vi "Save_Raw_data.vi"(4 "Add to Block Header":string, 7 "append to file? (new file:F)":bool, 8 "Block Timings":T1) -> (2 "Block Header":string)   [LabVIEW 2021]
uses:
  Controls/Block_start_and_end.ctl
  Acquisition/PWA/PWAtasksGLOBAL.vi
  Globals/Meas_global.vi
  Globals/Constants_global.vi
  Globals/LDA_global.vi
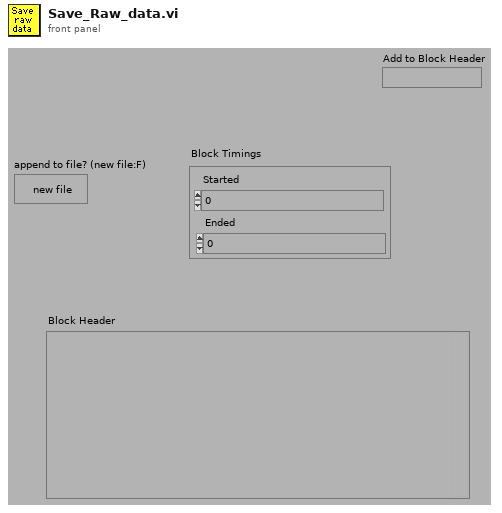
[diagram p1: front panel]
types:
  T1 = typedef "Block_start_and_end.ctl" = cluster{"Started":dbl, "Ended":dbl}
  T2 = cluster{"scale multiplier":dbl, "scale offset":dbl, "Length":i32, "I16 data":i16[], "Sampling rate (Hz)":dbl}
  T3 = typedef "Analysis_info_cluster.ctl" = cluster{"Colour":u32, "Inst type":T4, "Inst name":string, "Symbol":string, "Code name":string, "Extra Info":string, "Inst Array":T5, "Extra Titles":string[], "Extra Values":string[], "U":dbl, "u^2":dbl, "u^3":dbl, "u^4":dbl, "Skew_u":dbl, "Kurt_u":dbl, "Sd Error in Mean":dbl, "% u'/U":dbl, "X":dbl, "Y":dbl, "Z":dbl, "Timescale integral Estimate":dbl, "Sd Error in Variance":dbl, "Calib File":path, "Calib Constants":dbl[], "Output Position":bool, "Stats":enum16{"None", "Basic", "Full"}, "Av Sampling Rate":dbl, "Av No of Samples":dbl, "Total Meas Time (s)":dbl, "ADAM Ch Name":string, "Max value":dbl, "Min value":dbl, "Req Sample Rate Hz":dbl, "Sync Delay Time (s)":dbl, "Ch No":i16, "Device":string, "Use Latest Calib":bool, "Port":string, "Metadata Ch Names":string[], "Metadata Ch Values":string[], "Label":string}
  T4 = typedef "Inst_type.ctl" = enum16{"Raw voltage", "Raw with zero offsetting", "Propeller anemometer", "Pressure Transducer", "Pitot-static tube", "Hot wire", "Cross wire 1", "Cross wire 2", "Generic Linear", "Generic Polynomial", "Generic BackPoly", "Fast FID", "Thermocouple", "Cold wire", "Pulsed Wire", "LDA Vel", "LDA Tran time", "LDA Arr time", "Microphone"}
  T5 = typedef "Instrument_Array.ctl" = enum16{"PWA", "LDA", "Analogue"}
  T6 = typedef "Time_Trace_Cluster.ctl" = cluster{"Weighting":dbl[], "Time (s)":dbl[], "Voltage":dbl[], "Eng Values":dbl[]}
  T7 = cluster{"scale multiplier":dbl, "scale offset":dbl}[]
  T8 = typedef "PWA_Data.ctl" = enum16{"No PWA Data", "One Ch PWA"}
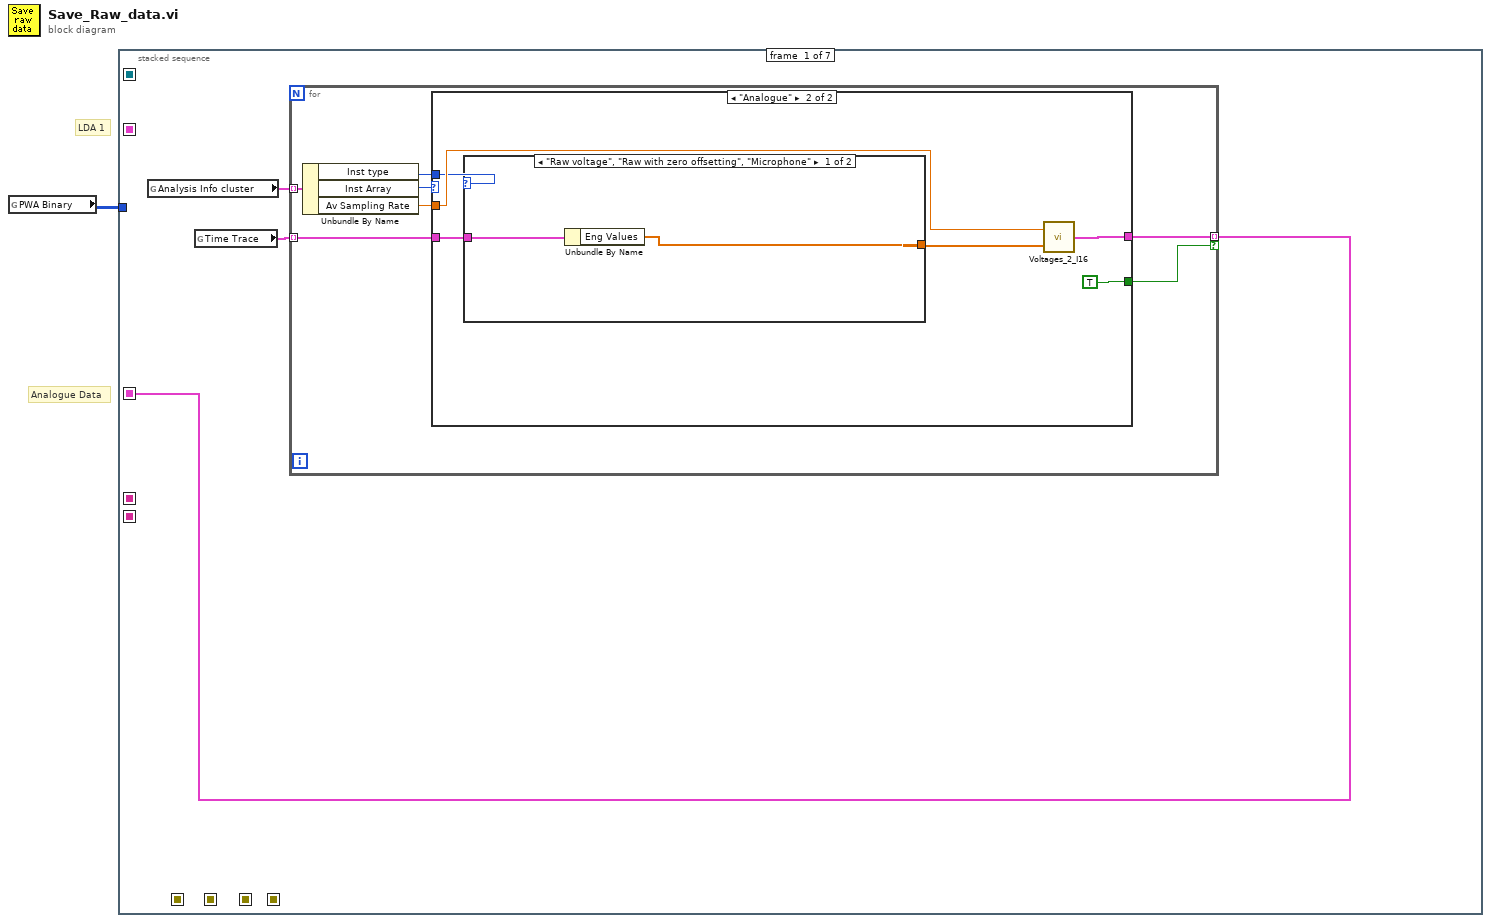
[diagram p0: block diagram]
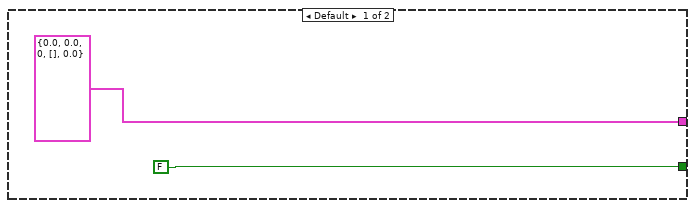
[diagram p2: hidden frame]
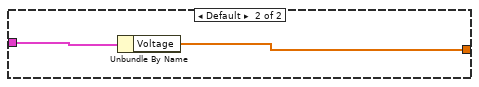
[diagram p3: hidden frame]
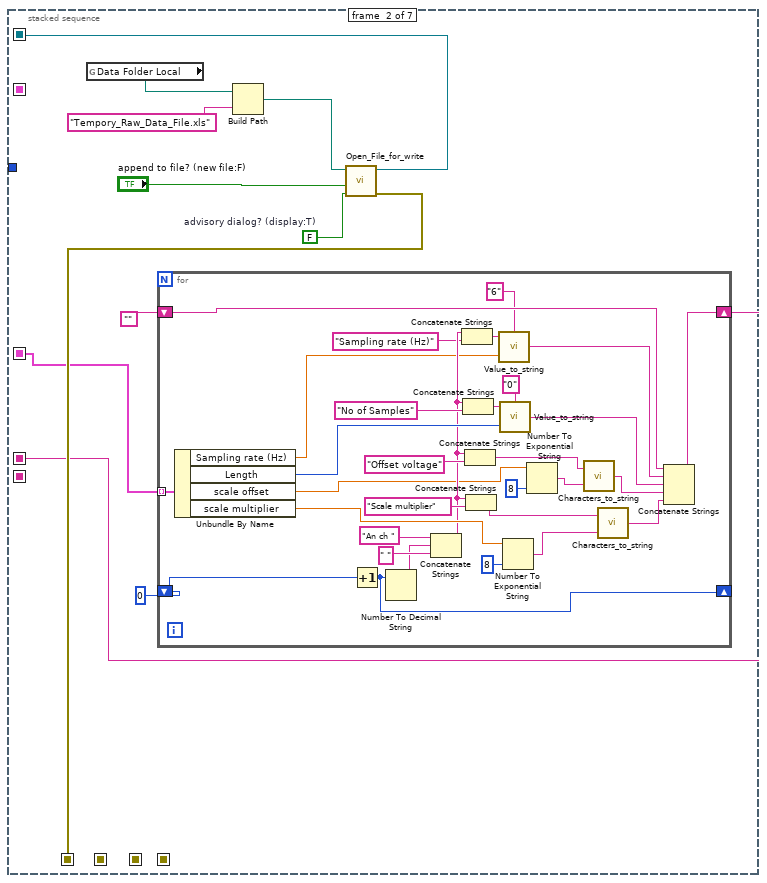
[diagram p4: hidden frame]
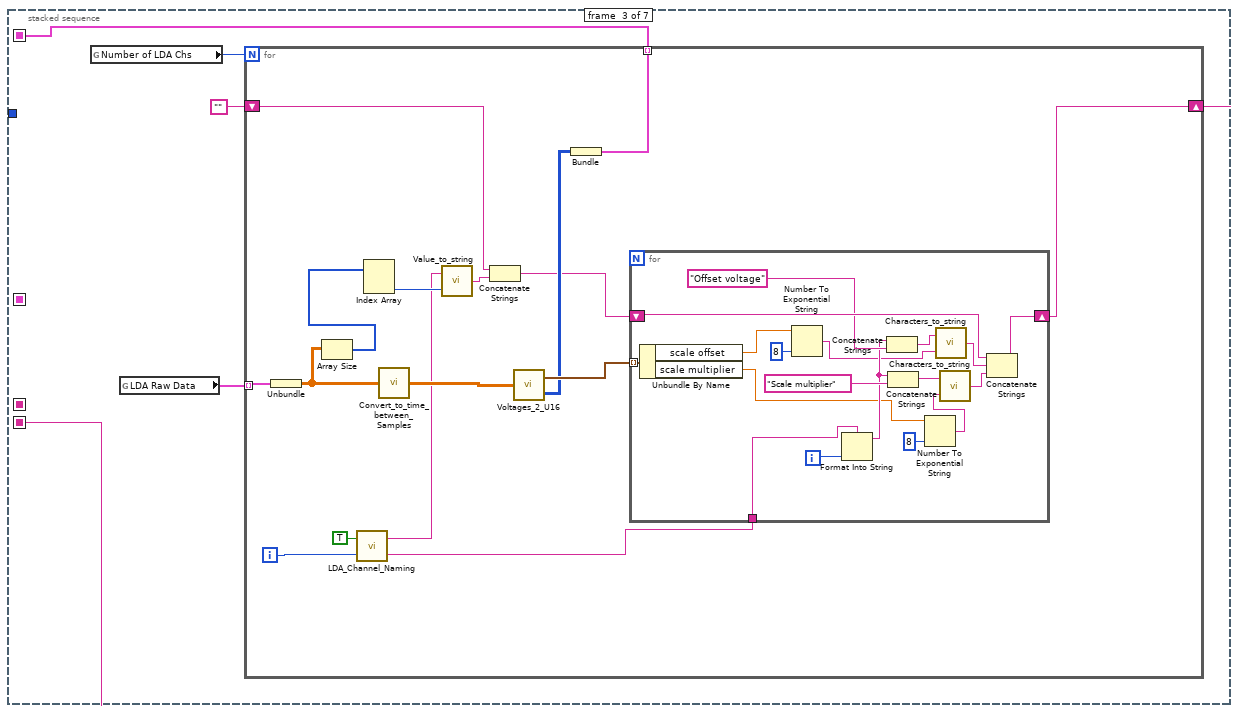
[diagram p5: hidden frame]
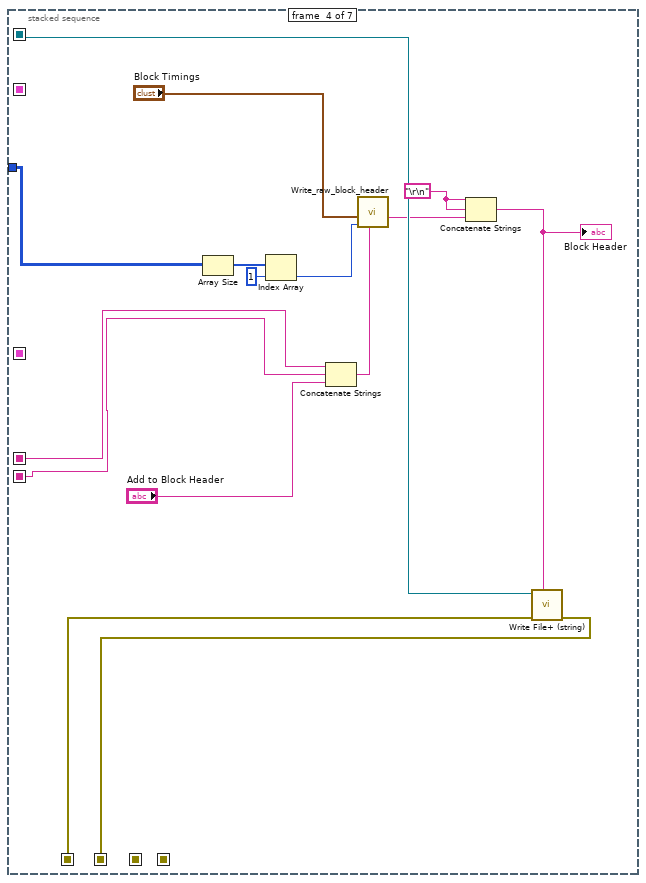
[diagram p6: hidden frame]
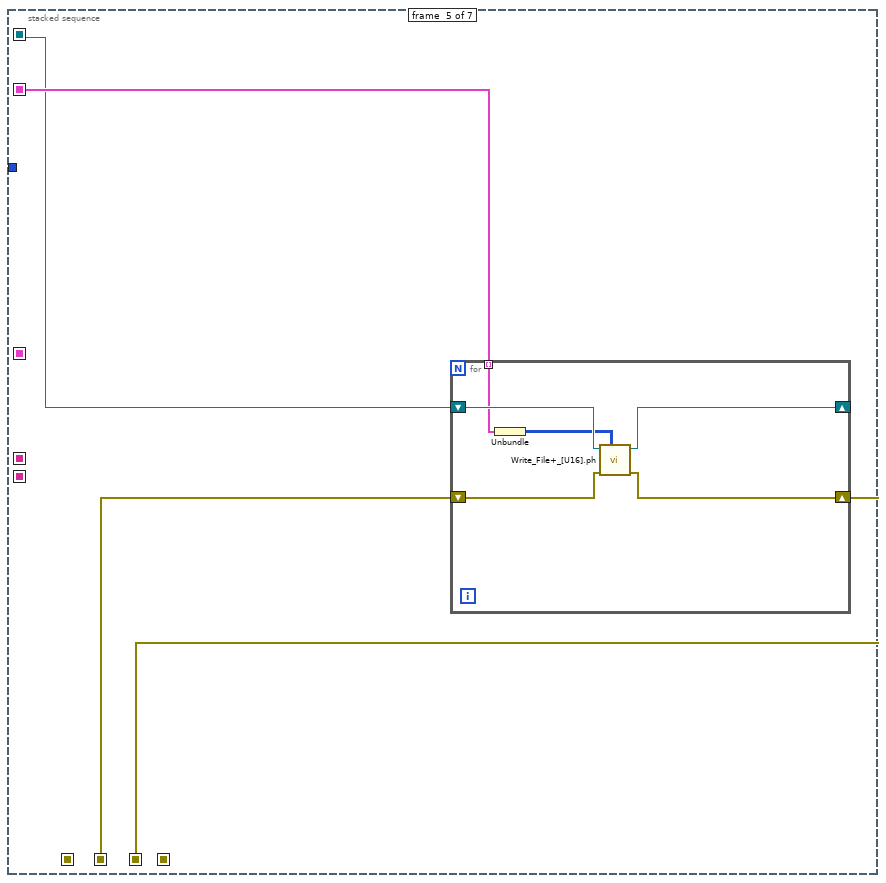
[diagram p7: hidden frame]
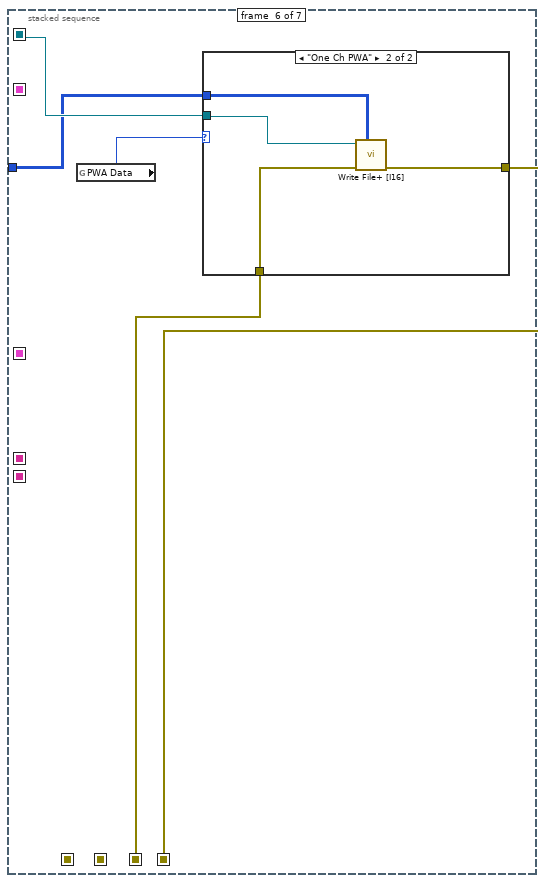
[diagram p8: hidden frame]
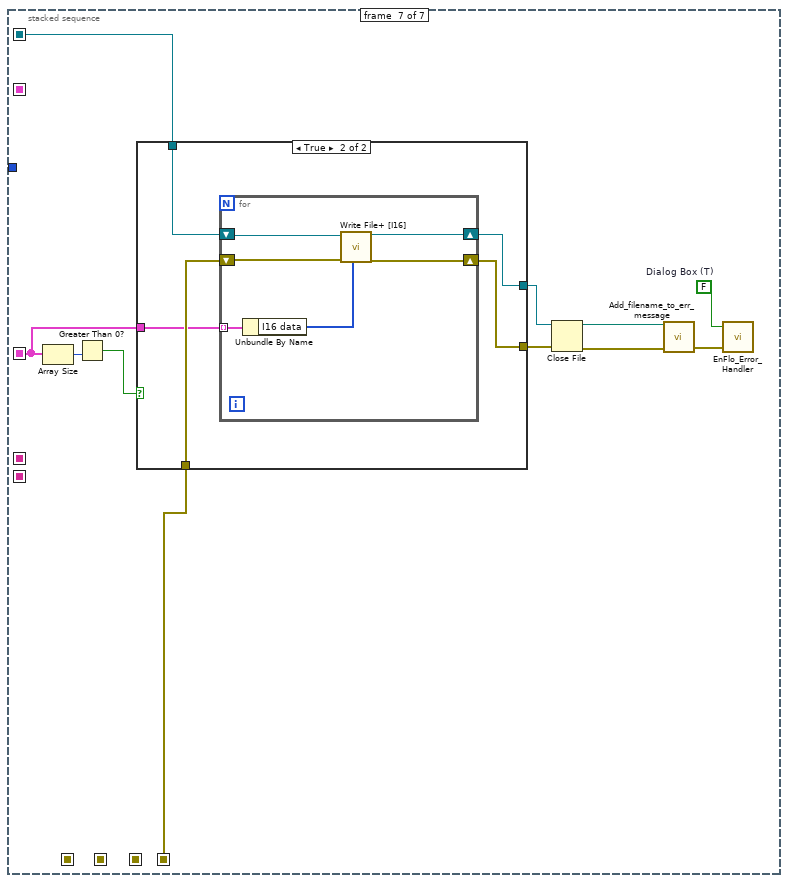
[diagram p10: hidden frame]
diagram:
  # "LDA 1"
  # "Analogue Data"
  n1 = global read "PWAtasksGLOBAL.vi" "PWA Binary"() -> (w1:i16[][])
  n2 = stacked-sequence {
    seq-local: [_ w34 _ _ _ _ _] -> [_ _ _ w119 w120 w133 w150]
    seq-local: [_ w33 _ _ _ _ _] -> [_ _ _ w118 _ _ _]
    seq-local: [_ _ _ w117 _ _ _] -> [_ _ _ _ w122 _ _]
    seq-local: [_ _ _ _ w121 _ _] -> [_ _ _ _ _ w132 _]
    seq-local: [_ _ _ _ _ w131 _] -> [_ _ _ _ _ _ w143]
    seq-local: [_ w25 _ _ _ _ _] -> [_ _ _ w106 _ _ _]
    seq-local: [_ _ w66 _ _ _ _] -> [_ _ _ _ w123 _ _]
    seq-local: [_ _ w67 _ _ _ _] -> [_ _ _ w105 _ _ _]
    seq-local: [w2 _ _ _ _ _ _] -> [_ w24 _ _ _ _ w140]
    tunnel: w1 -> [_ _ _ w111 _ w130 _]
    frame #0 {
      n3 = global read "Meas_global.vi" "Analysis Info cluster"() -> (w4:T3[])
      n4 = global read "Meas_global.vi" "Time Trace"() -> (w3:T6[])
      n5 = for {
        tunnel: w4 -> [w11] mode=indexing
        tunnel: w3 -> [w9] mode=indexing
        tunnel: [w8] -> w2 mode=indexing if=w7
        n6 = Unbundle By Name(w11) -> ("Inst type"=w5:T4, "Inst Array"=w10:T5, "Av Sampling Rate"=w6:dbl)
        n7 = case shown="\"Analogue\"" w10 {
          tunnel: w9 -> [_ w19]
          tunnel: [T2 {"scale multiplier"=0.0, "scale offset"=0.0, "Length"=0, "I16 data"=[], "Sampling rate (Hz)"=0.0} ("Channel Data") w15] -> w8
          tunnel: [FALSE TRUE] -> w7
          tunnel: w6 -> [_ w16]
          tunnel: w5 -> [_ w14]
          frame Default {
          }
          frame "Analogue" {
            n8 = case shown="\"Raw voltage\", \"Raw with zero offsetting\", \"Microphone\"" w14 {
              tunnel: w19 -> [w21 w23]
              tunnel: [w20 w22] -> w18
              frame "Raw voltage", "Raw with zero offsetting", "Microphone" {
                n9 = Unbundle By Name(w21) -> ("Eng Values"=w20:dbl[])
              }
              frame Default {
                n10 = Unbundle By Name(w23) -> ("Voltage"=w22:dbl[])
              }
            }
            n11 = call "Voltages_2_I16.vi"("Voltages"=w18, "Av Sampling Rate"=w16) -> ("Channel Data"=w15:T2)
          }
        }
      }
    }
    frame #1 {
      w32 = FALSE  # advisory dialog? (display:T)
      n12 = global read "Constants_global.vi" "Data Folder Local"() -> (w31:path)
      n13 = for {
        shift-right: [w65] -> w25
        shift-left: "" -> [w43]
        shift-right: [w63] -> _
        shift-left: 0 -> [w64]
        tunnel: w24 -> [w53] mode=indexing
        n14 = Unbundle By Name(w53) -> ("Sampling rate (Hz)"=w44:dbl, "Length"=w49:i32, "scale offset"=w37:dbl, "scale multiplier"=w52:dbl)
        n15 = Increment(x=w64) -> (x+1=w63:i32)
        n16 = Number To Decimal String(number=w63) -> (decimal integer string=w58:string)  [unwired: 1 out]
        n17 = Concatenate Strings("An ch ", w58, " ") -> (w46:string)
        n18 = Concatenate Strings(w46, "Sampling rate (Hz)" ("string")) -> (w47:string)
        n19 = Concatenate Strings(w46, "No of Samples") -> (w51:string)
        n20 = Concatenate Strings(w46, "Offset voltage") -> (w38:string)
        n21 = Concatenate Strings(w46, "Scale multiplier") -> (w55:string)
        n22 = call "Value_to_string.vi"("precision"="6", "Value"=w44, "Label for value"=w47) -> ("Output string"=w42:string)
        n23 = call "Value_to_string.vi"("precision"="0", "Value"=w49, "Label for value"=w51) -> ("Output string"=w41:string)
        n24 = Number To Exponential String(number=w52, precision (6)=i16 8) -> (E-format string=w54:string)  [unwired: 2 out]
        n25 = Number To Exponential String(number=w37, precision (6)=i16 8) -> (E-format string=w39:string)  [unwired: 2 out]
        n26 = call "Characters_to_string.vi"("Characters to write"=w39, "Label for characters"=w38) -> ("Output string"=w36:string)  [unwired: 1 in]
        n27 = call "Characters_to_string.vi"("Characters to write"=w54, "Label for characters"=w55) -> ("Output string"=w56:string)  [unwired: 1 in]
        n28 = Concatenate Strings(w43, w42, w41, w36, w56) -> (w65:string)
      }
      n29 = Build Path(base path=w31, name or relative path="Tempory_Raw_Data_File.xls") -> (appended path=w29:path)
      n30 = call "Open_File_for_write.vi"("advisory dialog? (display:T)"=w32, "append to file? (new file:F)"="append to file? (new file:F)", "file path"=w29) -> ("error out"=w33:errorcluster, "refnum"=w34:refnum<file>)  [unwired: 7 out]
    }
    frame #2 {
      n31 = global read "LDA_global.vi" "Number of LDA Chs"() -> (w70:i32)
      n32 = global read "LDA_global.vi" "LDA Raw Data"() -> (w69:cluster{dbl[][]}[])
      n33 = for {
        N: w70 -> [_]
        tunnel: w69 -> [w82] mode=indexing
        shift-right: [w81] -> w67
        shift-left: "" -> [w74]
        tunnel: [w80] -> w66 mode=indexing
        i -> [w84]
        n34 = Unbundle(w82) -> (w77:dbl[][])
        n35 = Array Size(array=w77) -> (size(s)=w76:i32[])
        n36 = call "LDA_Channel_Naming.vi"("Numeric"=w84, "After May 2019"=TRUE) -> ("Channel Name"=w83:string, "No of Samples"=w72:string)
        n37 = Index Array(array=w76) -> (element #2=w79:i32)  [unwired: 2 in, 1 out]
        n38 = call "Convert_to_time_between_Samples.vi"("LDA 1st Group in"=w77) -> ("LDA 1st Group out"=w85:dbl[][])
        n39 = call "Value_to_string.vi"("Value"=w79, "Label for value"=w72) -> ("Output string"=w75:string)  [unwired: 1 in]
        n40 = Concatenate Strings(w74, w75) -> (w73:string)
        n41 = call "Voltages_2_U16.vi"("Voltages"=w85) -> ("Scale and Offset"=w86:T7, "U16 data"=w78:u16[][])
        n42 = Bundle("U16 data"=w78) -> (w80:cluster{"U16 data":u16[][]})  [unwired: 1 in]
        n43 = for {
          shift-right: [w103] -> w81
          shift-left: w73 -> [w104]
          tunnel: w86 -> [w96] mode=indexing
          tunnel: w83 -> [w87]
          i -> [w94]
          n44 = Unbundle By Name(w96) -> ("scale offset"=w90:dbl, "scale multiplier"=w93:dbl)
          n45 = Number To Exponential String(number=w90, precision (6)=i16 8) -> (E-format string=w89:string)  [unwired: 2 out]
          n46 = Format Into String(format string=w87, w94) -> (resulting string=w95:string)  [unwired: 2 in, 1 out]
          n47 = Concatenate Strings(w95, "Offset voltage") -> (w92:string)
          n48 = Concatenate Strings(w95, "Scale multiplier") -> (w98:string)
          n49 = Number To Exponential String(number=w93, precision (6)=i16 8) -> (E-format string=w97:string)  [unwired: 2 out]
          n50 = call "Characters_to_string.vi"("Characters to write"=w89, "Label for characters"=w92) -> ("Output string"=w88:string)  [unwired: 1 in]
          n51 = call "Characters_to_string.vi"("Characters to write"=w97, "Label for characters"=w98) -> ("Output string"=w99:string)  [unwired: 1 in]
          n52 = Concatenate Strings(w104, w88, w99) -> (w103:string)
        }
      }
    }
    frame #3 {
      w114 = "\r\n"
      n53 = Array Size(array=w111) -> (size(s)=w112:i32[])
      n54 = Index Array(array=w112, index=1) -> (element=w110:i32)
      n55 = Concatenate Strings(w106, w105, "Add to Block Header") -> (w107:string)
      n56 = call "Write_raw_block_header.vi"("Block Timings"="Block Timings", "No of PWA samples"=w110, "Add to Block Header"=w107) -> ("Output string"=w115:string)  [unwired: 2 in]
      n57 = Concatenate Strings(w114, w114, w115) -> (w109:string)
      "Block Header" <- w109
      n58 = call <vilib>:"Write File+ (string).vi"("string"=w109, "error in (no error)"=w118, "refnum"=w119) -> ("error out"=w117:errorcluster)  [unwired: 2 in, 4 out]
    }
    frame #4 {
      n59 = for {
        shift-right: [w126] -> _
        shift-left: w120 -> [w127]
        shift-right: [w128] -> w121
        shift-left: w122 -> [w129]
        tunnel: w123 -> [w125] mode=indexing
        n60 = Unbundle(w125) -> ("U16 data"=w124:u16[][])
        n61 = call "Write_File+_[U16].ph.vi"("2D array"=w124, "error in (no error)"=w129, "refnum"=w127) -> ("error out"=w128:errorcluster, "dup refnum"=w126:refnum<file>)  [unwired: 3 in, 4 out]
      }
    }
    frame #5 {
      n62 = global read "Meas_global.vi" "PWA Data"() -> (w134:T8)
      n63 = case shown="\"One Ch PWA\"" w134 {
        tunnel: w130 -> [_ w137]
        tunnel: w133 -> [_ w136]
        tunnel: w132 -> [w135 w139]
        tunnel: [w135 w138] -> w131
        frame "No PWA Data" {
        }
        frame "One Ch PWA" {
          n64 = call <vilib>:"Write File+ [I16].vi"("2D array"=w137, "error in (no error)"=w139, "refnum"=w136) -> ("error out"=w138:errorcluster)  [unwired: 3 in, 5 out]
        }
      }
    }
    frame #6 {
      w148 = FALSE  # Dialog Box (T)
      n65 = Array Size(array=w140) -> (size(s)=w142:i32)
      n66 = Greater Than 0?(x=w142) -> (x > 0?=w141:bool)
      n67 = case shown="True" w141 {
        tunnel: w150 -> [w152 w154]
        tunnel: w143 -> [w151 w157]
        tunnel: [w151 w156] -> w147
        tunnel: [w152 w155] -> w146
        tunnel: w140 -> [_ w153]
        frame False {
        }
        frame True {
          n68 = for {
            shift-right: [w162] -> w156
            shift-left: w157 -> [w163]
            shift-right: [w161] -> w155
            shift-left: w154 -> [w160]
            tunnel: w153 -> [w159] mode=indexing
            n69 = Unbundle By Name(w159) -> ("I16 data"=w158:i16[])
            n70 = call <vilib>:"Write File+ [I16].vi"("1D array"=w158, "error in (no error)"=w163, "refnum"=w160) -> ("error out"=w162:errorcluster, "dup refnum"=w161:refnum<file>)  [unwired: 3 in, 4 out]
          }
        }
      }
      n71 = Close File(refnum=w146, error in=w147) -> (path=w144:path, error out=w145:errorcluster)
      n72 = call "Add_filename_to_err_message.vi"("error in (no error)"=w145, "Path"=w144) -> ("error out"=w149:errorcluster)
      n73 = call "EnFlo_Error_Handler.vi"("error in (no error)"=w149, "Dialog Box (F)"=w148) -> ()  [unwired: 1 in, 3 out]
    }
  }
